vi "CAEN_HVSystem.get i attribute.vi"(0 "i ref in":refnum<vi>, 5 "error in (no error)":errorcluster) -> (14 "i ref out":refnum<vi>, 16 "i attribute":T1 {"FrontPanOut"."FrontPanOut" format="%.0b"; "FrontPanIn"."FrontPanIn" format="%.0b"; "GenSignCfg"."GenSignCfg" format="%.0b"}, 19 "error out":errorcluster)   [LabVIEW 2014, in "CAEN_HVSystem.lvlib"]
doc: "Gets the i attribute data of an object.\n\nLicense Agreement for this software:\n\nCopyright (C)\nGesellschaft für Schwerionenforschung, GSI\nPlanckstr. 1\n64291 Darmstadt\nGermany\n\nContact: D.Beck@gsi.de \n\nThis program is free software; you can redistribute it and/or modify it under the terms of the GNU General Public License as published by the Free Software Foundation; either version 2 of the license, or (at your option) any later version.\n\nThis program is distributed in the hope that it will be useful, but WITHOUT ANY WARRANTY; without even the implied warranty of MERCHANTABILITY or FITNESS FOR A PARTICULAR PURPOSE. See the GNU General License for more details (http://www.gnu.org).\n\nGesellschaft für Schwerionenforschung, GSI\nPlanckstr. 1, 64291 Darmstadt, Germany\nFor all questions and ideas contact: M.Richter@gsi.de, H.Brand@gsi.de or D.Beck@gsi.de.\nLast update: 17-JUN-2004"
uses:
  CAEN_HVSystem.lvlib
  CAEN_HVSystem.i attribute.ctl
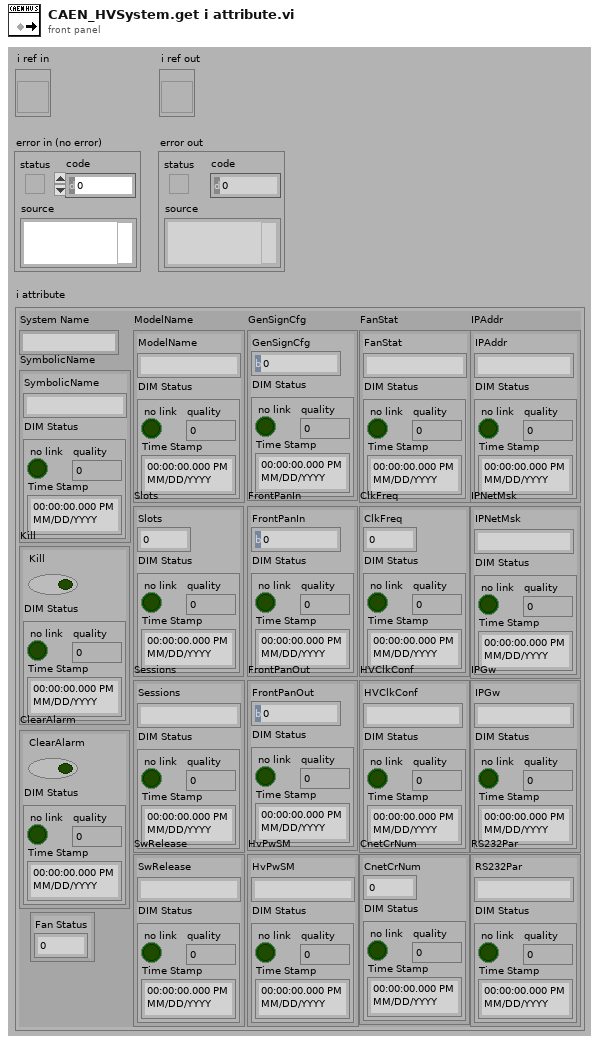
[diagram p1: front panel]
types:
  T1 = typedef "CAEN_HVSystem.lvlib/CAEN_HVSystem.i attribute.ctl" = cluster{"System Name":string, "DIM Service IDs":cluster{"Fan Status":i32}, "SymbolicName":cluster{"SymbolicName":string, "DIM Status":cluster{"no link":bool, "quality":i32, "Time Stamp":timestamp}}, "ModelName":cluster{"ModelName":string, "DIM Status":cluster{"no link":bool, "quality":i32, "Time Stamp":timestamp}}, "Slots":cluster{"Slots":i16, "DIM Status":cluster{"no link":bool, "quality":i32, "Time Stamp":timestamp}}, "Kill":cluster{"Kill":bool, "DIM Status":cluster{"no link":bool, "quality":i32, "Time Stamp":timestamp}}, "ClearAlarm":cluster{"ClearAlarm":bool, "DIM Status":cluster{"no link":bool, "quality":i32, "Time Stamp":timestamp}}, "Sessions":cluster{"Sessions":string, "DIM Status":cluster{"no link":bool, "quality":i32, "Time Stamp":timestamp}}, "SwRelease":cluster{"SwRelease":string, "DIM Status":cluster{"no link":bool, "quality":i32, "Time Stamp":timestamp}}, "GenSignCfg":cluster{"GenSignCfg":i16, "DIM Status":cluster{"no link":bool, "quality":i32, "Time Stamp":timestamp}}, "FrontPanIn":cluster{"FrontPanIn":i16, "DIM Status":cluster{"no link":bool, "quality":i32, "Time Stamp":timestamp}}, "FrontPanOut":cluster{"FrontPanOut":i16, "DIM Status":cluster{"no link":bool, "quality":i32, "Time Stamp":timestamp}}, "HvPwSM":cluster{"HvPwSM":string, "DIM Status":cluster{"no link":bool, "quality":i32, "Time Stamp":timestamp}}, "FanStat":cluster{"FanStat":string, "DIM Status":cluster{"no link":bool, "quality":i32, "Time Stamp":timestamp}}, "ClkFreq":cluster{"ClkFreq":i16, "DIM Status":cluster{"no link":bool, "quality":i32, "Time Stamp":timestamp}}, "HVClkConf":cluster{"HVClkConf":string, "DIM Status":cluster{"no link":bool, "quality":i32, "Time Stamp":timestamp}}, "CnetCrNum":cluster{"CnetCrNum":i16, "DIM Status":cluster{"no link":bool, "quality":i32, "Time Stamp":timestamp}}, "IPAddr":cluster{"IPAddr":string, "DIM Status":cluster{"no link":bool, "quality":i32, "Time Stamp":timestamp}}, "IPNetMsk":cluster{"IPNetMsk":string, "DIM Status":cluster{"no link":bool, "quality":i32, "Time Stamp":timestamp}}, "IPGw":cluster{"IPGw":string, "DIM Status":cluster{"no link":bool, "quality":i32, "Time Stamp":timestamp}}, "RS232Par":cluster{"RS232Par":string, "DIM Status":cluster{"no link":bool, "quality":i32, "Time Stamp":timestamp}}}
  T2 = enum16{"SetAttribute", "GetAttribute", "CreateAttribute", "DestroyAttribute", "DestroyAllAtributes"}
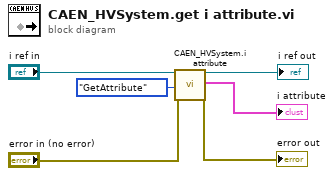
[diagram p0: block diagram]
diagram:
  n1 = call "CAEN_HVSystem.i attribute.vi"("VI Refnum"="i ref in", "Action"=T2."GetAttribute", "error in (no error)"="error in (no error)") -> ("VI Refnum out"=→"i ref out":refnum<vi>, "CLASS.i attribute out"=→"i attribute":T1, "error out"=→"error out":errorcluster)  [unwired: 14 in]
